vi "Extract2Dslices-xy-zx-zy.vi"(10 "xyz pos":u16[](array[numeric]), 11 "zyx":u16[][][](array[numeric])) -> (1 "zy":u16[][](array[numeric]), 2 "zx":u16[][](array[numeric]), 3 "yx":u16[][](array[numeric]))   [LabVIEW 2024]
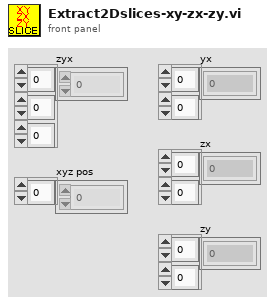
[diagram p1: front panel]
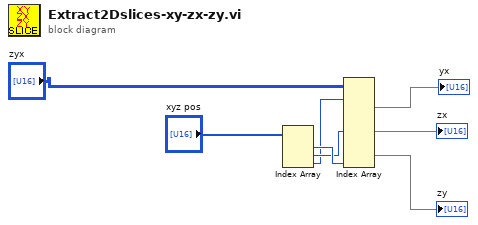
[diagram p0: block diagram]
diagram:
  n1 = Index Array(array="xyz pos") -> (element #1=w5:u16, element #2=w4:u16, element #3=w3:u16)  [unwired: 3 in]
  n2 = Index Array(array="zyx", index (dim 0) #1=w3, index (dim 1) #2=w4, index (dim 2) #3=w5) -> (element #1=→"yx":u16[][], element #2=→"zx":u16[][], element #3=→"zy":u16[][])  [unwired: 6 in]
